vi "DSCSV2SVRef.vi"(1 "Shared Variable Control":refnum<k21>) -> (0 "shared variable refnum":refnum<k21>)   [LabVIEW 2009, in "MoAgSy_Base.lvlib"]
uses:
  MoAgSy_Base.lvlib
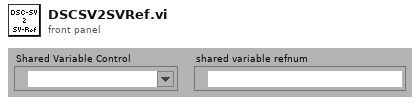
[diagram p1: front panel]
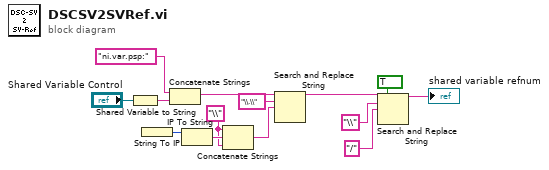
[diagram p0: block diagram]
diagram:
  w1 = "\\" ("string")
  n1 = Shared Variable to String(1:"Shared Variable Control") -> (0:w13:string)
  n2 = String To IP() -> (0:w7:u32)  [unwired: 1 in]
  n3 = Concatenate Strings("ni.var.psp:" ("string"), w13) -> (w6:string)
  n4 = IP To String(2:w7) -> (0:w4:string)  [unwired: 1 in]
  n5 = Concatenate Strings(w1, w4, w1) -> (w2:string)
  n6 = Search and Replace String(input string=w6, search string="\\.\\", replace string=w2) -> (result string=w3:string)  [unwired: 5 in, 3 out]
  n7 = Search and Replace String(replace all?=TRUE ("replace all? (F)"), input string=w3, search string="\\", replace string="/" ("replace string (\"\")")) -> (result string=→"shared variable refnum":string)  [unwired: 4 in, 3 out]
